vi "Read Tree Tag.vi"(8 "error in (no error)":errorcluster, 11 "Data Item in":refnum<class "Data Item.lvclass">) -> (0 "error out":errorcluster, 2 "Tree Tag":string, 3 "Data Item out":refnum<class "Data Item.lvclass">)   [LabVIEW 2020, in "VILab.lvlib" / "Data Item.lvclass"]
uses:
  Data Item.lvclass
  Data Item.lvclass/Data Item.ctl
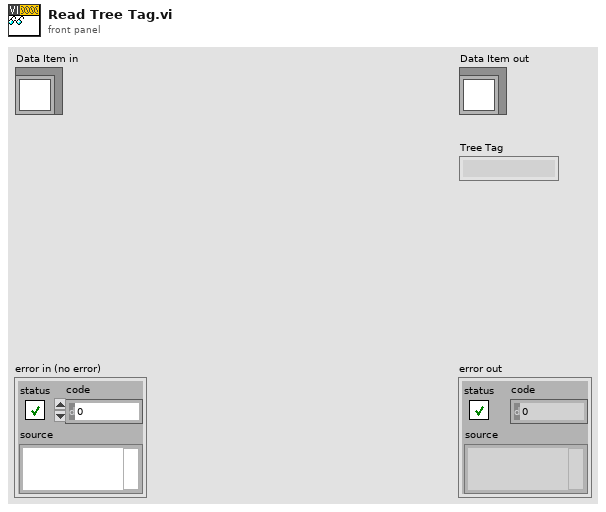
[diagram p1: front panel]
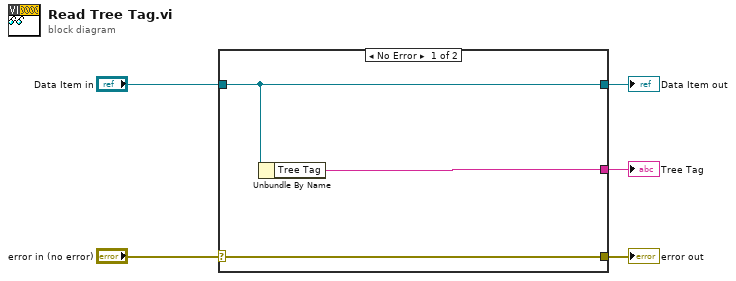
[diagram p0: block diagram]
diagram:
  n1 = case shown="No Error" "error in (no error)" {
    selector: "error in (no error)" -> [w8 w9]
    tunnel: [w8 w9] -> w4
    tunnel: [w7 w10] -> w2
    tunnel: "Data Item in" -> [w7 w10]
    tunnel: [w6 _] -> w1
    frame No Error {
      n2 = Unbundle By Name(w7) -> ("Tree Tag"=w6:string)
    }
    frame Error {
    }
  }
  "error out" <- w4
  "Data Item out" <- w2
  "Tree Tag" <- w1
